vi "FT Controls Change.vi"(8 "error in (no error)":errorcluster, 9 "F/T Ctrls Cluster Variant":variant, 11 "Rigol DG822 Sine in":refnum<class "Rigol DG822 Sine.lvclass">) -> (0 "error out":errorcluster, 1 "New F/T Ctrls Cluster Variant":variant, 3 "Rigol DG822 Sine out":refnum<class "Rigol DG822 Sine.lvclass">)   [LabVIEW 2021, in "Rigol DG822 UI.lvlib" / "Rigol DG822 Sine.lvlib" / "Rigol DG822 Sine.lvclass"]
uses:
  Rigol DG822 Sine.lvclass
  Rigol DG822 UI/lib/controls.llb/FT Controls Cluster.ctl
  Rigol DG822 Sine.lvclass/Rigol DG822 Sine.ctl
  General/Files/lvlibp/Actors.lvlibp/Actors/Actors/Actors.lvclass
  D:/LabVIEW/General/Files/lvlibp/Actors.lvlibp/Actors/Actors/Actors.lvclass
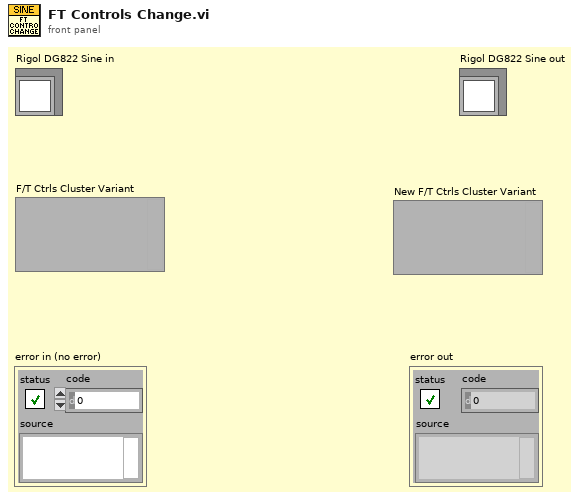
[diagram p1: front panel]
types:
  T1 = cluster{"Freq/Period":bool, "Ampl/HighL":bool, "Offset/LowL":bool}
  T2 = typedef "FT Controls Cluster.ctl" = cluster{"Freq/Period":bool, "Ampl/HighL":bool, "Offset/LowL":bool, "Duty/Width":bool}
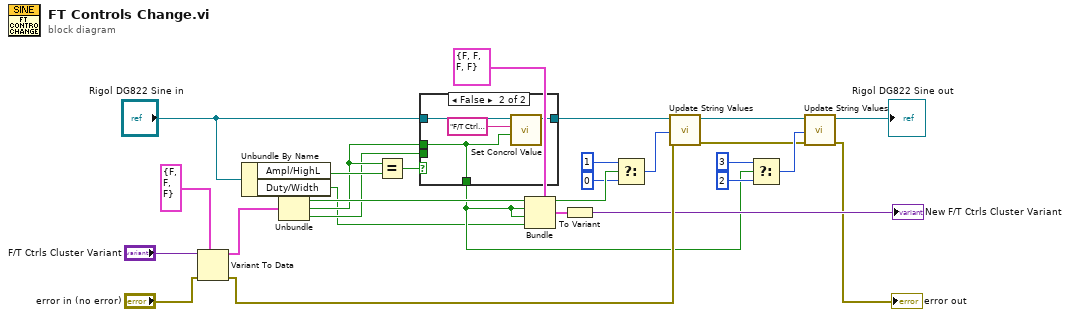
[diagram p0: block diagram]
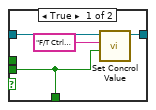
[diagram p2: hidden frame]
diagram:
  n1 = Variant To Data(error in="error in (no error)", type=T1 {"Freq/Period"=FALSE, "Ampl/HighL"=FALSE, "Offset/LowL"=FALSE} ("NewVal"), Variant="F/T Ctrls Cluster Variant") -> (data=w27:T1, error out=w24:errorcluster)
  n2 = Unbundle By Name("Rigol DG822 Sine in") -> ("Ampl/HighL"=w4:bool, "Duty/Width"=w1:bool)
  n3 = Unbundle(w27) -> ("Freq/Period"=w22:bool, "Ampl/HighL"=w3:bool, "Offset/LowL"=w2:bool)
  n4 = Equal?(x=w3, y=w4) -> (x = y?=w26:bool)
  n5 = case shown="False" w26 {
    tunnel: [w31 w35] -> w15
    tunnel: "Rigol DG822 Sine in" -> [w29 w33]
    tunnel: w2 -> [w28 _]
    tunnel: w3 -> [_ w32]
    tunnel: [w28 w32] -> w8
    frame True {
      n6 = call "Set Concrol Value.vi"("Value"=w28, "Control Label"="F/T Ctrls.Ampl/HighL", "Actors in"=w29) -> ("Actors out"=w31:refnum<class "Rigol DG822 Sine.lvclass">)  [unwired: 7 in, 1 out]
    }
    frame False {
      n7 = call "Set Concrol Value.vi"("Value"=w32, "Control Label"="F/T Ctrls.Offset/LowL", "Actors in"=w33) -> ("Actors out"=w35:refnum<class "Rigol DG822 Sine.lvclass">)  [unwired: 7 in, 1 out]
    }
  }
  n8 = Bundle(cluster=T2 {"Freq/Period"=FALSE, "Ampl/HighL"=FALSE, "Offset/LowL"=FALSE, "Duty/Width"=FALSE} ("F/T Ctrls"), "Freq/Period"=w22, "Ampl/HighL"=w8, "Offset/LowL"=w8, "Duty/Width"=w1) -> (w21:T2)
  n9 = To Variant(anything=w21) -> (Variant=→"New F/T Ctrls Cluster Variant":variant)
  n10 = Select(t=u16 1 ("Type"), s=w22, f=u16 0) -> (s? t:f=w18:u16)
  n11 = call-dynamic "Update String Values.vi"("error in (no error)"=w24, "Type"=w18, "Rigol DG822 Sine in"=w15) -> ("error out"=w11:errorcluster, "Rigol DG822 Sine out"=w12:refnum<class "Rigol DG822 Sine.lvclass">)  [unwired: 7 in]
  n12 = Select(t=u16 3 ("Type"), s=w8, f=u16 2) -> (s? t:f=w13:u16)
  n13 = call-dynamic "Update String Values.vi"("error in (no error)"=w11, "Type"=w13, "Rigol DG822 Sine in"=w12) -> ("error out"=→"error out":errorcluster, "Rigol DG822 Sine out"=→"Rigol DG822 Sine out":refnum<class "Rigol DG822 Sine.lvclass">)  [unwired: 7 in]
